vi "LEDSubVi.vi"(2 "Thing in":refnum<class "Thing.lvclass">, 3 "Numeric":i32, 4 "ValueToWrite":bool) -> (1 "WritenValue":bool)   [LabVIEW 2016]
uses:
  <vilib>/National Instruments/IoT Education Toolkit Beta/TW API/Thing.lvclass
  <vilib>/National Instruments/IoT Education Toolkit Beta/TW API/TW_SetPropertyValue_Boolean_Public.vi
  <vilib>/National Instruments/IoT Education Toolkit Beta/TW API/Properties.lvclass
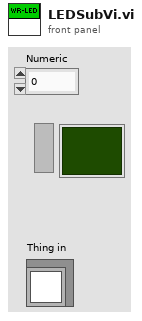
[diagram p1: front panel]
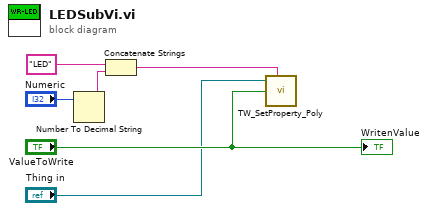
[diagram p0: block diagram]
diagram:
  n1 = Number To Decimal String(number="Numeric") -> (decimal integer string=w5:string)  [unwired: 1 in]
  n2 = Concatenate Strings("LED", w5) -> (w2:string)
  n3 = call-poly <vilib>:"TW_SetProperty_Poly.vi"("Thing in"="Thing in", "Property name"=w2, "Value"="ValueToWrite") -> ()  [unwired: 3 in, 2 out]
  "WritenValue" <- "ValueToWrite"
